vi "rethinkdb_query_base.vi"(6 "timeout ms (10000)":i32=10000, 7 "query_token":u64=1 format="%016x", 8 "error in (no error)":errorcluster, 10 "query":string="[1,\"foo\",{}]", 11 "rethinkdb in":refnum<k5>) -> (0 "error out":errorcluster, 2 "response_json":string, 3 "rethinkdb out":refnum<k5>, 4 "remaining_data":string, 5 "response_token":u64)   [LabVIEW 2017]
panel:
  out "response_length":i32
  out "data_read":string
  out "data_written":string
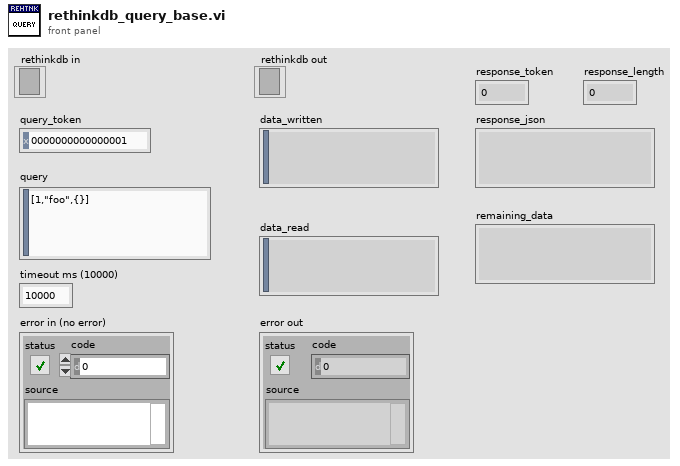
[diagram p1: front panel]
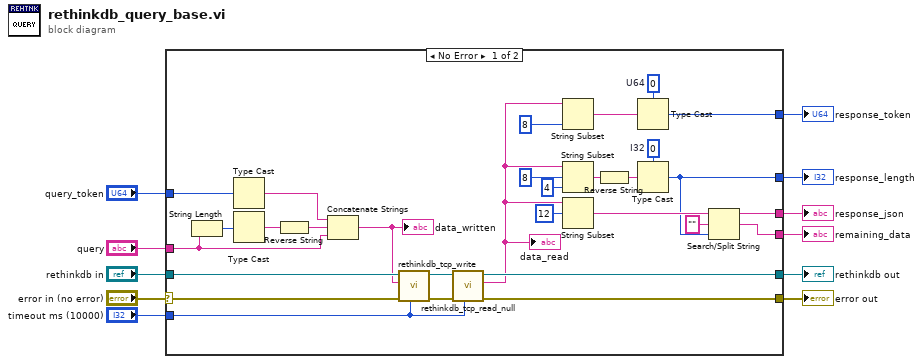
[diagram p0: block diagram]
diagram:
  n1 = case shown="No Error" "error in (no error)" {
    selector: "error in (no error)" -> [w41 w43]
    tunnel: "rethinkdb in" -> [w40 w42]
    tunnel: [w39 w43] -> w9
    tunnel: [w38 w42] -> w8
    tunnel: "query_token" -> [w37 _]
    tunnel: "query" -> [w34 _]
    tunnel: "timeout ms (10000)" -> [w32 _]
    tunnel: [w24 _] -> w4
    tunnel: [w15 _] -> w3
    tunnel: [w13 _] -> w2
    tunnel: [w12 _] -> w1
    frame No Error {
      w20 = 0  # I32
      w25 = u64 0  # U64
      n2 = String Length(string=w34) -> (length=w30:i32)
      n3 = Type Cast(x=w37) -> (*(type *) &x=w31:string)  [unwired: 1 in]
      n4 = Type Cast(x=w30) -> (*(type *) &x=w36:string)  [unwired: 1 in]
      n5 = Reverse String(1:w36) -> (0:w35:string)
      n6 = Concatenate Strings(w31, w35, w34) -> (w33:string)
      "data_written" <- w33
      n7 = call "rethinkdb_tcp_write.vi"("timeout ms (10000)"=w32, "error in (no error)"=w41, "data in"=w33, "rethinkdb in"=w40) -> ("error out"=w29:errorcluster, "rethinkdb out"=w28:refnum<k5>)  [unwired: 5 in, 1 out]
      n8 = call "rethinkdb_tcp_read_null.vi"("timeout ms (10000)"=w32, "error in (no error)"=w29, "rethinkdb in"=w28) -> ("error out"=w39:errorcluster, "data out"=w17:string, "rethinkdb out"=w38:refnum<k5>)  [unwired: 6 in]
      "data_read" <- w17
      n9 = String Subset(string=w17, length (rest)=8 ("length (rest)")) -> (substring=w26:string)  [unwired: 1 in]
      n10 = String Subset(string=w17, offset (0)=8 ("length (rest)"), length (rest)=4 ("length (rest)")) -> (substring=w21:string)
      n11 = String Subset(string=w17, offset (0)=12) -> (substring=w16:string)  [unwired: 1 in]
      n12 = Reverse String(1:w21) -> (0:w19:string)
      n13 = Type Cast(type=w25, x=w26) -> (*(type *) &x=w24:u64)
      n14 = Type Cast(type=w20, x=w19) -> (*(type *) &x=w15:i32)
      n15 = Search/Split String(string=w16, search string/char (-)="", offset (0)=w15) -> (substring before match=w13:string, match + rest of string=w12:string)  [unwired: 1 out]
    }
    frame Error {
    }
  }
  "error out" <- w9
  "rethinkdb out" <- w8
  "response_token" <- w4
  "response_length" <- w3
  "response_json" <- w2
  "remaining_data" <- w1
